vi "Get current direction.vi"(8 "error in (no error)":errorcluster, 11 "Lifter_motor in":refnum<class "Lifter_motor.lvclass">) -> (0 "error out":errorcluster, 2 "Direction":bool, 3 "Lifter_motor out":refnum<class "Lifter_motor.lvclass">)   [LabVIEW 2019, in "Lifter_motor.lvclass"]
uses:
  Lifter_motor.lvclass
  Lifter_motor.lvclass/Lifter_motor.ctl
  TCP Class/LifterTCP.lvclass
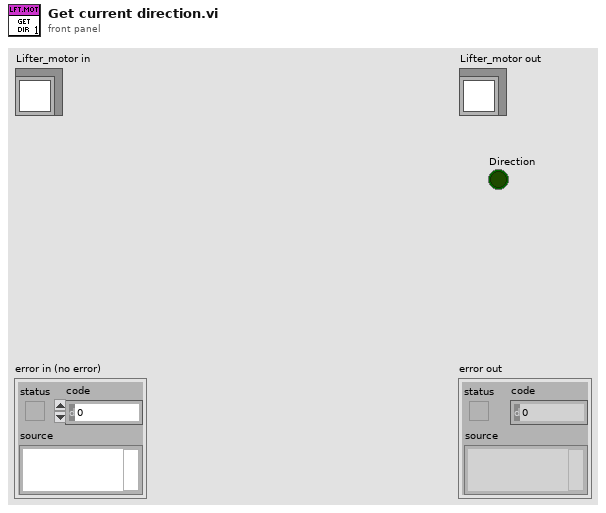
[diagram p1: front panel]
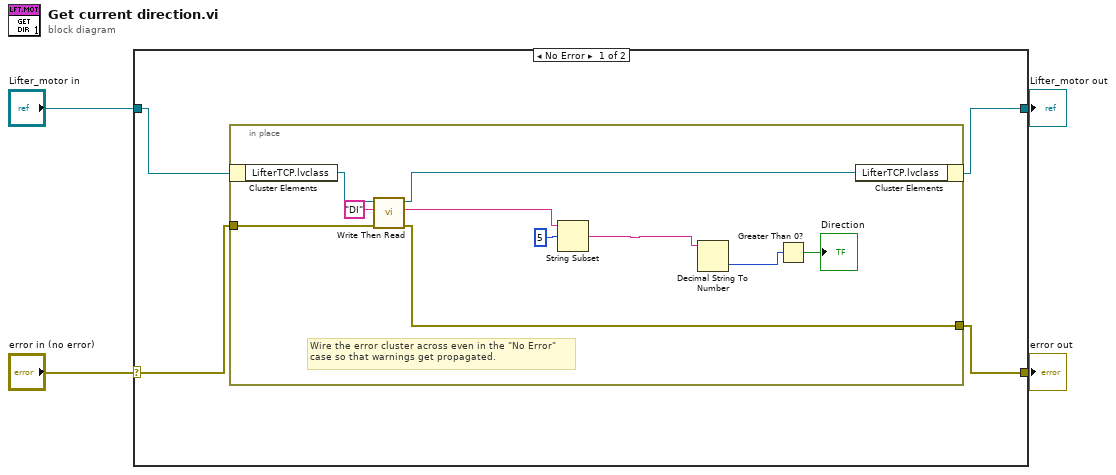
[diagram p0: block diagram]
diagram:
  n1 = case shown="No Error" "error in (no error)" {
    selector: "error in (no error)" -> [w8 w20]
    tunnel: [w7 w20] -> w3
    tunnel: [w6 w19] -> w1
    tunnel: "Lifter_motor in" -> [w5 w19]
    frame No Error {
      # "Wire the error cluster across even in the \"No Error\"\ncase so that warnings get propagated."
      n2 = in-place {
        in-place-border: w8 -> [w17]
        in-place-border: [w13] -> w7
        n3 = in-place-cluster #1(w5) -> ("LifterTCP.lvclass"=w18:refnum<class "LifterTCP.lvclass">)
        n4 = call "Write Then Read.vi"("error in (no error)"=w17, "Parameter 1"="DI", "LifterTCP in"=w18) -> ("error out"=w13:errorcluster, "Read Data"=w15:string, "LifterTCP out"=w14:refnum<class "LifterTCP.lvclass">)  [unwired: 6 in]
        n5 = String Subset(string=w15, offset (0)=5) -> (substring=w11:string)  [unwired: 1 in]
        n6 = Decimal String To Number(string=w11) -> (number=w10:i32)  [unwired: 2 in, 1 out]
        n7 = Greater Than 0?(x=w10) -> (x > 0?=→"Direction":bool)
        n8 = in-place-cluster #1("LifterTCP.lvclass"=w14) -> (w6:refnum<class "Lifter_motor.lvclass">)
      }
    }
    frame Error {
    }
  }
  "error out" <- w3
  "Lifter_motor out" <- w1
